vi "read_stimulus_alignment_command_h5.vi"(11 "Path":path) -> (0 "error out":errorcluster, 3 "stimulus":i32[](array[numeric]))   [LabVIEW 2015]
uses:
  <vilib>/addons/h5labview2/file/H5Fmode.ctl
  <vilib>/addons/h5labview2/base/lib_path.vi
  <vilib>/addons/h5labview2/base/H5Equery.vi
  <vilib>/addons/h5labview2/base/hid_t.ctl
  <vilib>/addons/h5labview2/dataset/H5Dread.llb/H5Dread.xnode
  <vilib>/addons/h5labview2/file/H5F.lvlib
  <vilib>/addons/h5labview2/group/H5G.lvlib
panel:
  out "Waveform Graph":i32[](graph)
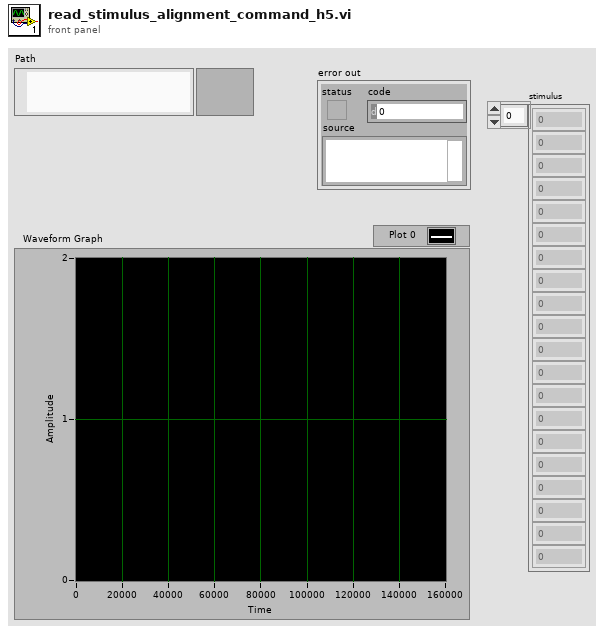
[diagram p1: front panel]
types:
  T1 = typedef "H5F.lvlib/H5Fmode.ctl" = enum16{"read-only", "read-write", "overwrite", "create new", "open or create"}
  T2 = typedef "hid_t.ctl" = i32
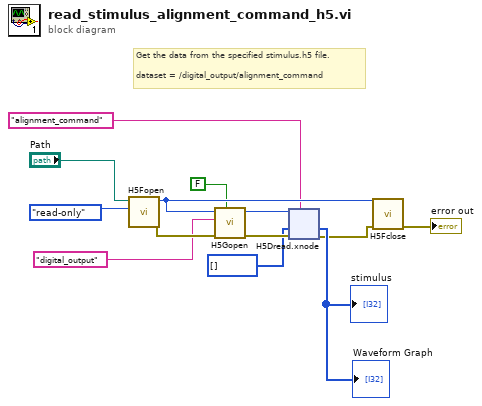
[diagram p0: block diagram]
diagram:
  # "Get the data from the specified stimulus.h5 file.\n\ndataset = /digital_output/alignment_command"
  n1 = call <vilib>:"H5Fopen.vi"("mode (read-only)"=H5Fmode."read-only" ("mode"), "path"="Path") -> ("error out"=w11:errorcluster, "ref out"=w12:T2)  [unwired: 8 in]
  n2 = call <vilib>:"H5Gopen.vi"("create? (F)"=FALSE, "error in (no error)"=w11, "name"="digital_output", "ref in"=w12) -> ("error out"=w9:errorcluster, "group out"=w5:T2)  [unwired: 6 in]
  n3 = xnode "H5Dread.xnode"("dataset name (this)"="alignment_command" ("name"), "error in (no error)"=w9, "default"=i32[] [] ("data"), "ref in"=w5) -> ("error out"=w1:errorcluster, "data"=→"stimulus" →"Waveform Graph":i32[])  [unwired: 2 in, 2 out]
  n4 = call <vilib>:"H5Fclose.vi"("error in (no error)"=w1, "ref"=w12) -> ("error out"=→"error out":errorcluster)  [unwired: 9 in]
